vi "Main-Calculate PSD by ACF or direct FFT.vi"() -> ()   [LabVIEW 2014]
uses:
  <vilib>/Utility/file.llb/Read From Spreadsheet File (DBL).vi
  <vilib>/Analysis/NI_AALBase.lvlib
  <vilib>/Analysis/NI_AALPro.lvlib
panel:
  out "Avg. Array":dbl[](array[numeric])
  out "Frequency,0 df,2df,...,(Hz)":dbl[][](array[numeric])
  out "PSD":dbl[][](array[numeric])
  in  "dx":dbl
  out "Array 3":dbl[](array[numeric])
  out "Array 2":dbl[](array[numeric])
  in  "# of avg":i32
  out "Array":dbl[](array[numeric])
  in  "dcenter of hist":dbl
  out "Axis":dbl[](array[numeric]) format="%0.2f"
  out "df":dbl
  in  "ACF length":i32=2130
  in  "Filter?":bool
  in  "left rank":i32=2
  in  "Tab Control":enum32{"Page 1", "Page 2", "Page 3", "Page 4"}(tab)
  out "Waveform Graph":dbl[](graph)
  out "XY Graph":T1(graph)
  out "XY Graph 2":T1(graph)
  out "XY Graph 3":cluster{"Avg. Array":dbl[], "Avg. Array":dbl[]}(graph)
  out "Fs":dbl
  in  "intervals":i32=5000
  in  "T=ACF method\nF=direct FT method":bool
  in  "file path (dialog if empty)":path=path "D:/OneDrive - NTU.gg/OT/OT data/YCC/20190524-/FA-S-2-4-m51-Ca/pFC/All useful traces.txt"
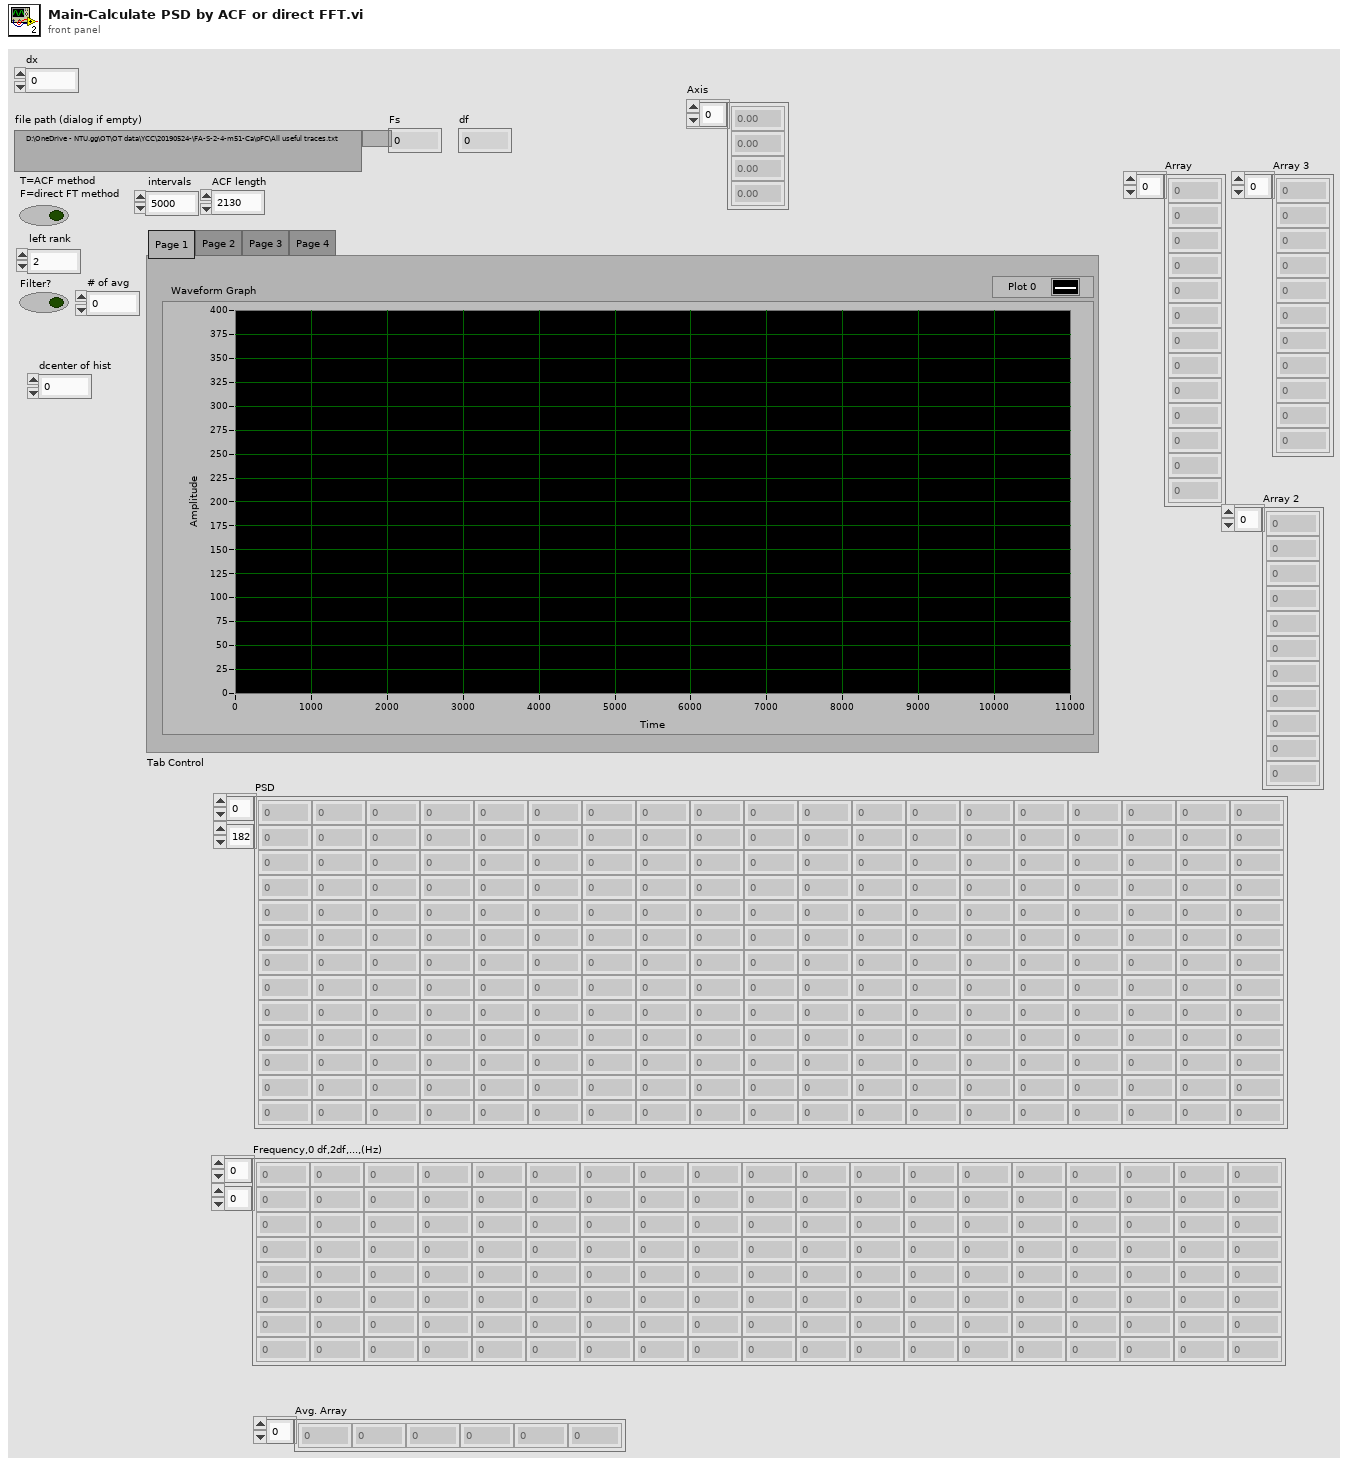
[diagram p1: front panel]
types:
  T1 = cluster{"Frequency,0 df,2df,...,(Hz)":dbl[], "PSD":dbl[]}
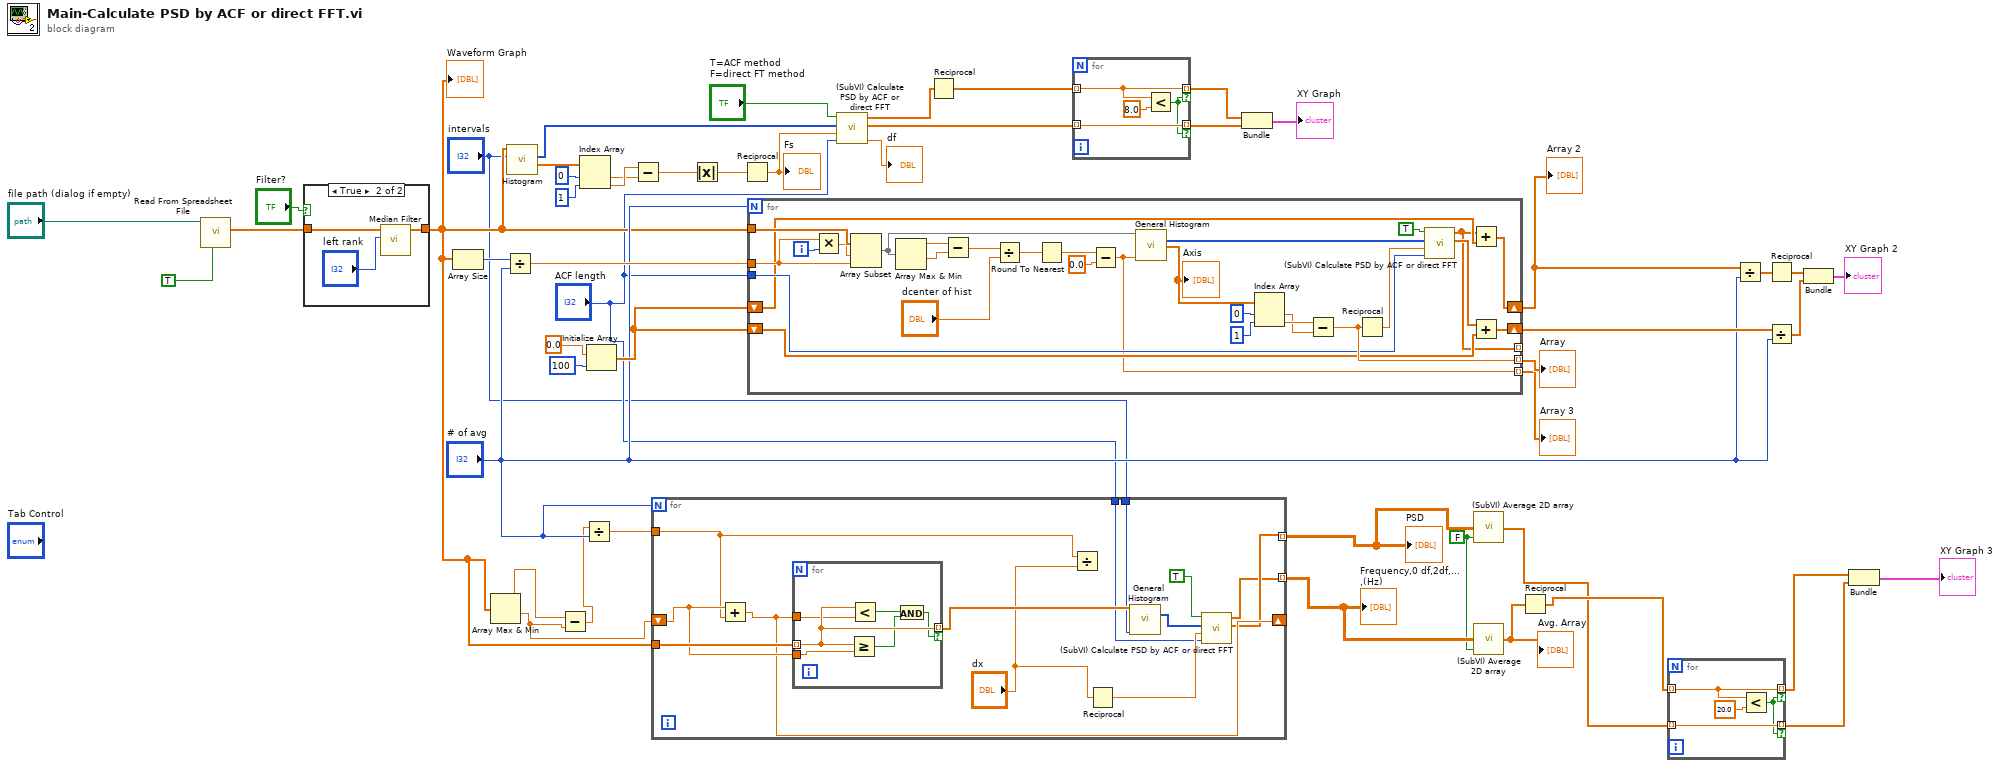
[diagram p0: block diagram]
diagram:
  w8 = FALSE ("Transpose?")
  n1 = call-poly <vilib>:"Read From Spreadsheet File.vi"("transpose (no:F)"=TRUE, "file path (dialog if empty)"="file path (dialog if empty)") -> ("first row"=w37:dbl[])  [unwired: 5 in, 4 out]
  n2 = case shown="True" "Filter?" {
    tunnel: w37 -> [w52 w55]
    tunnel: [w52 w54] -> w14
    frame False {
    }
    frame True {
      n3 = call <vilib>:"Median Filter.vi"("left rank"="left rank", "X"=w55) -> ("Filtered X"=w54:dbl[])  [unwired: 8 in, 1 out]
    }
  }
  "Waveform Graph" <- w14
  n4 = Array Size(array=w14) -> (size(s)=w29:i32)
  n5 = Array Max & Min(array=w14) -> (max value=w17:dbl, min value=w13:dbl)  [unwired: 2 out]
  n6 = Divide(x=w29, y="# of avg") -> (x/y=w28:dbl)
  n7 = call <vilib>:"Histogram.vi"("intervals"="intervals", "X"=w14) -> ("X Values"=w48:dbl[], "Histogram: h(x)"=w40:i32[])  [unwired: 6 in, 2 out]
  n8 = Subtract(x=w17, y=w13) -> (x-y=w15:dbl)
  n9 = Index Array(array=w48, index #1=0 ("index"), index #2=1 ("index")) -> (element #1=w44:dbl, element #2=w45:dbl)
  n10 = Divide(x=w15, y="# of avg") -> (x/y=w12:dbl)
  n11 = Initialize Array(0.0 ("element"), 100 ("dimension size")) -> (w18:dbl[])
  n12 = Subtract(x=w45, y=w44) -> (x-y=w43:dbl)
  n13 = for {
    N: "# of avg" -> [_]
    tunnel: w14 -> [w68]
    tunnel: w12 -> [w65]
    shift-right: [w59] -> _
    shift-left: w13 -> [w67]
    tunnel: "ACF length" -> [w60]
    tunnel: [w58] -> w10 mode=indexing
    tunnel: [w57] -> w9 mode=indexing
    tunnel: "intervals" -> [w56]
    n14 = Add(x=w67, y=w65) -> (x+y=w59:dbl)
    n15 = for {
      tunnel: w68 -> [w74] mode=indexing
      tunnel: [w74] -> w66 mode=indexing if=w71
      tunnel: w67 -> [w70]
      tunnel: w59 -> [w69]
      n16 = Greater Or Equal?(x=w74, y=w70) -> (x >= y?=w72:bool)
      n17 = Less?(x=w74, y=w69) -> (x < y?=w73:bool)
      n18 = And(x=w73, y=w72) -> (x .and. y?=w71:bool)
    }
    n19 = Divide(x=w65, y="dx") -> ()  [unwired: 1 out]
    n20 = Reciprocal(x="dx") -> (1/x=w61:dbl)
    n21 = call <vilib>:"General Histogram.vi"("X"=w66, "# bins"=w56) -> ("Histogram"=w63:i32[])  [unwired: 9 in, 4 out]
    n22 = call "(SubVI) Calculate PSD by ACF or direct FFT.vi"("ACF length"=w60, "Fs"=w61, "Data"=w63, "T=ACF method\nF=direct FT method"=TRUE ("T=ACF method\nF=direct FT method")) -> ("PSD"=w58:dbl[], "Frequency,0 df,2df,...,(Hz)"=w57:dbl[])  [unwired: 2 in, 2 out]
  }
  "PSD" <- w10
  "Frequency,0 df,2df,...,(Hz)" <- w9
  n23 = Absolute Value(x=w43) -> (abs(x)=w42:dbl)
  n24 = Reciprocal(x=w42) -> (1/x=w41:dbl)
  "Fs" <- w41
  n25 = for {
    N: "# of avg" -> [_]
    tunnel: w14 -> [w96]
    tunnel: [w84] -> w30 mode=indexing
    tunnel: w28 -> [w88]
    tunnel: "ACF length" -> [w82]
    shift-right: [w80] -> w27
    shift-left: w18 -> [w81]
    shift-right: [w77] -> w26
    shift-left: w18 -> [w78]
    tunnel: [w76] -> _ mode=indexing
    tunnel: [w75] -> w20 mode=indexing
    i -> [w89]
    n26 = Multiply(x=w88, y=w89) -> (x*y=w87:dbl)
    n27 = Array Subset(array=w96, index=w87, length=w88) -> (w95:dbl[])
    n28 = Array Max & Min(array=w95) -> (max value=w100:dbl, min value=w99:dbl)  [unwired: 2 out]
    n29 = Subtract(x=w100, y=w99) -> (x-y=w98:dbl)
    n30 = Divide(x=w98, y="dcenter of hist") -> (x/y=w93:dbl)
    n31 = Round To Nearest(number=w93) -> (nearest integer value=w92:dbl)
    n32 = Subtract(x=w92, y=0.0) -> (x-y=w75:dbl)
    n33 = call <vilib>:"General Histogram.vi"("X"=w95, "# bins"=w75) -> ("Histogram"=w86:i32[], "Axis"=w103:dbl[])  [unwired: 9 in, 3 out]
    "Axis" <- w103
    n34 = Index Array(array=w103, index #1=0 ("index"), index #2=1 ("index")) -> (element #1=w90:dbl, element #2=w91:dbl)
    n35 = Subtract(x=w91, y=w90) -> (x-y=w84:dbl)
    n36 = Reciprocal(x=w84) -> (1/x=w83:dbl)
    n37 = call "(SubVI) Calculate PSD by ACF or direct FFT.vi"("ACF length"=w82, "Fs"=w83, "Data"=w86, "T=ACF method\nF=direct FT method"=TRUE ("T=ACF method\nF=direct FT method")) -> ("PSD"=w79:dbl[], "Frequency,0 df,2df,...,(Hz)"=w76:dbl[])  [unwired: 2 in, 2 out]
    n38 = Add(x=w76, y=w81) -> (x+y=w80:dbl[])
    n39 = Add(x=w79, y=w78) -> (x+y=w77:dbl[])
  }
  "Array" <- w30
  "Array 2" <- w27
  "Array 3" <- w20
  n40 = call "(SubVI) Calculate PSD by ACF or direct FFT.vi"("ACF length"="ACF length", "Fs"=w41, "Data"=w40, "T=ACF method\nF=direct FT method"="T=ACF method\nF=direct FT method") -> ("df"=→"df":dbl, "PSD"=w34:dbl[], "Frequency,0 df,2df,...,(Hz)"=w38:dbl[])  [unwired: 2 in, 1 out]
  n41 = Reciprocal(x=w38) -> (1/x=w35:dbl[])
  n42 = for {
    tunnel: w35 -> [w106] mode=indexing
    tunnel: w34 -> [w105] mode=indexing
    tunnel: [w106] -> w32 mode=indexing if=w104
    tunnel: [w105] -> w33 mode=indexing if=w104
    n43 = Less?(x=w106, y=8.0) -> (x < y?=w104:bool)
  }
  n44 = Bundle(w32, w33) -> (→"XY Graph":cluster{dbl[], dbl[]})  [unwired: 1 in]
  n45 = call "(SubVI) Average 2D array.vi"("Transpose?"=w8, "Array"=w10) -> ("Avg. Array"=w5:dbl[])  [unwired: 3 in]
  n46 = call "(SubVI) Average 2D array.vi"("Transpose?"=w8, "Array"=w9) -> ("Avg. Array"=w7:dbl[])  [unwired: 3 in]
  "Avg. Array" <- w7
  n47 = Reciprocal(x=w7) -> (1/x=w6:dbl[])
  n48 = for {
    tunnel: w6 -> [w110] mode=indexing
    tunnel: w5 -> [w109] mode=indexing
    tunnel: [w110] -> w4 mode=indexing if=w108
    tunnel: [w109] -> w3 mode=indexing if=w108
    n49 = Less?(x=w110, y=20.0) -> (x < y?=w108:bool)
  }
  n50 = Divide(x=w27, y="# of avg") -> (x/y=w25:dbl[])
  n51 = Reciprocal(x=w25) -> (1/x=w24:dbl[])
  n52 = Divide(x=w26, y="# of avg") -> (x/y=w23:dbl[])
  n53 = Bundle(w24, w23) -> (→"XY Graph 2":cluster{dbl[], dbl[]})  [unwired: 1 in]
  n54 = Bundle(w4, w3) -> (→"XY Graph 3":cluster{dbl[], dbl[]})  [unwired: 1 in]
